vi "LCR_PlotHelper.vi"(5 "Y-Axis":T3, 7 "X-Axis":T3, 9 "Data_IN":T1={"Value"=0.0, "GUI Data Cluster"={"SBR"=0}, "Timing"={"Last Operation"=0.0, "Stop @ T"=FALSE, "Delta T Log"=FALSE, "End T"=0.0, "Delta T"=0.0, "Last Temp"=0.0}, "Measurements"=[], "Hardware"={"VNA TCP Port"=5025, "Global T VAR"="", "Global B VAR"=""}} {"GUI Data Cluster"."SBR" format="%08b"}, 11 "Graph REF":refnum<vi>) -> (0 "Graph Out":cluster{"Variant X":dbl, "Variant Y":dbl}[](array[cluster]), 1 "Data_Out":T1={"Value"=0.0, "GUI Data Cluster"={"SBR"=0}, "Timing"={"Last Operation"=0.0, "Stop @ T"=FALSE, "Delta T Log"=FALSE, "End T"=0.0, "Delta T"=0.0, "Last Temp"=0.0}, "Measurements"=[], "Hardware"={"VNA TCP Port"=5025, "Global T VAR"="", "Global B VAR"=""}} {"GUI Data Cluster"."SBR" format="%08b"})   [LabVIEW 2021]
uses:
  Plotting-Axis.ctl
  Data_Cluster.ctl
  Measurement_Cluster.ctl
  82b2c7e2-1130-4631-9edb-692d0da541f7.vi
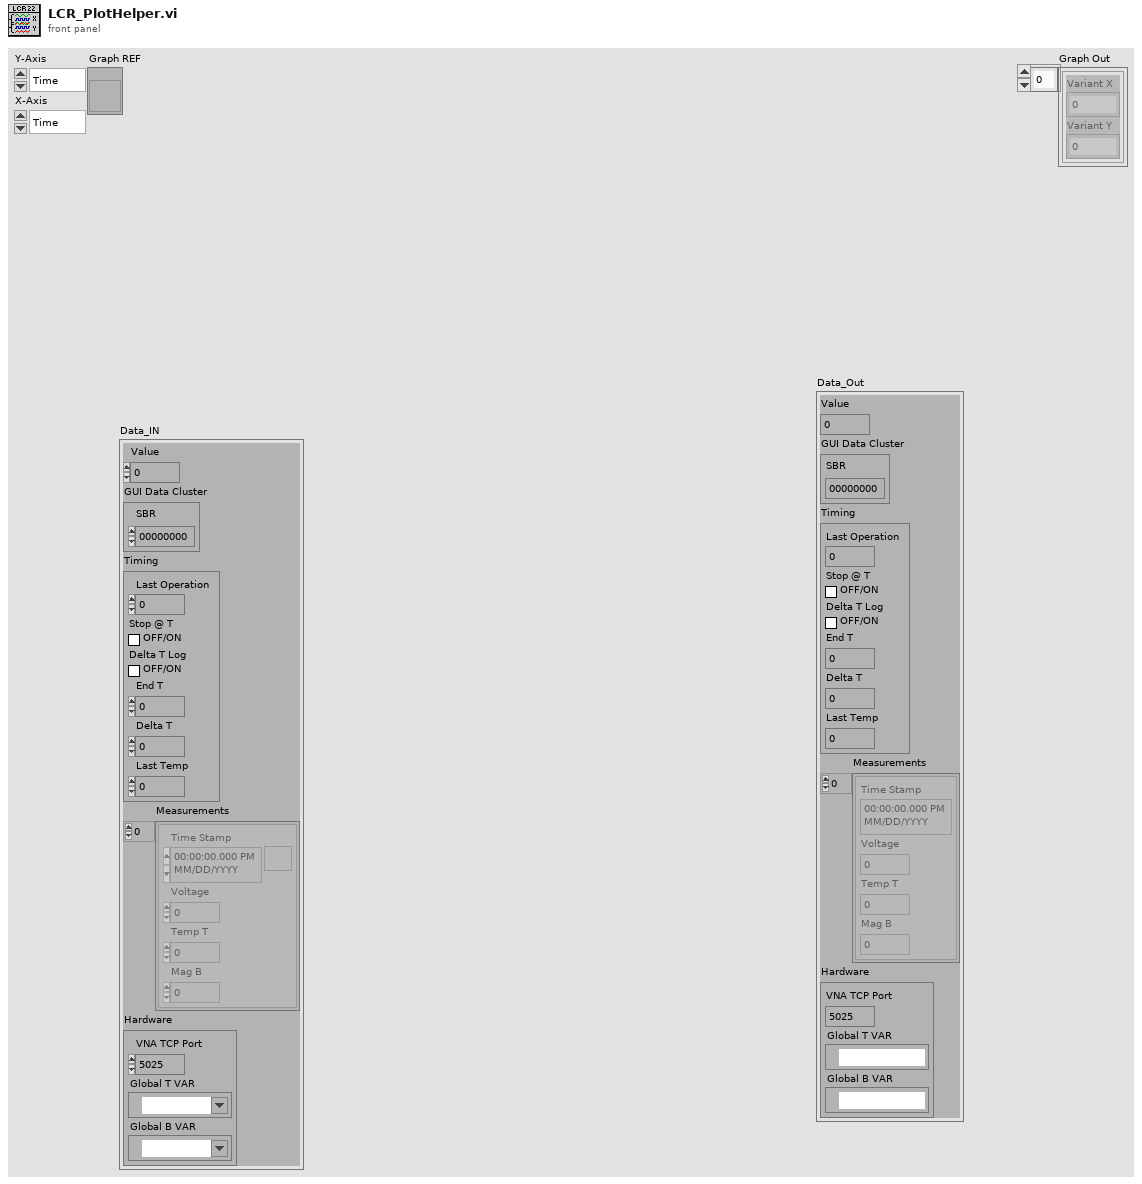
[diagram p1: front panel]
types:
  T1 = typedef "Data_Cluster.ctl" = cluster{"Value":dbl, "GUI Data Cluster":cluster{"SBR":u16}, "Timing":cluster{"Last Operation":dbl, "Stop @ T":bool, "Delta T Log":bool, "End T":dbl, "Delta T":dbl, "Last Temp":dbl}, "Measurements":T2[], "Hardware":cluster{"VNA TCP Port":i32, "Global T VAR":refnum<k21>, "Global B VAR":refnum<k21>}}
  T2 = typedef "Measurement_Cluster.ctl" = cluster{"Time Stamp":timestamp, "Voltage":dbl, "Temp T":dbl, "Mag B":dbl}
  T3 = typedef "Plotting-Axis.ctl" = enum16{"Time", "Temperature A", "Temperature B", "Voltage"}
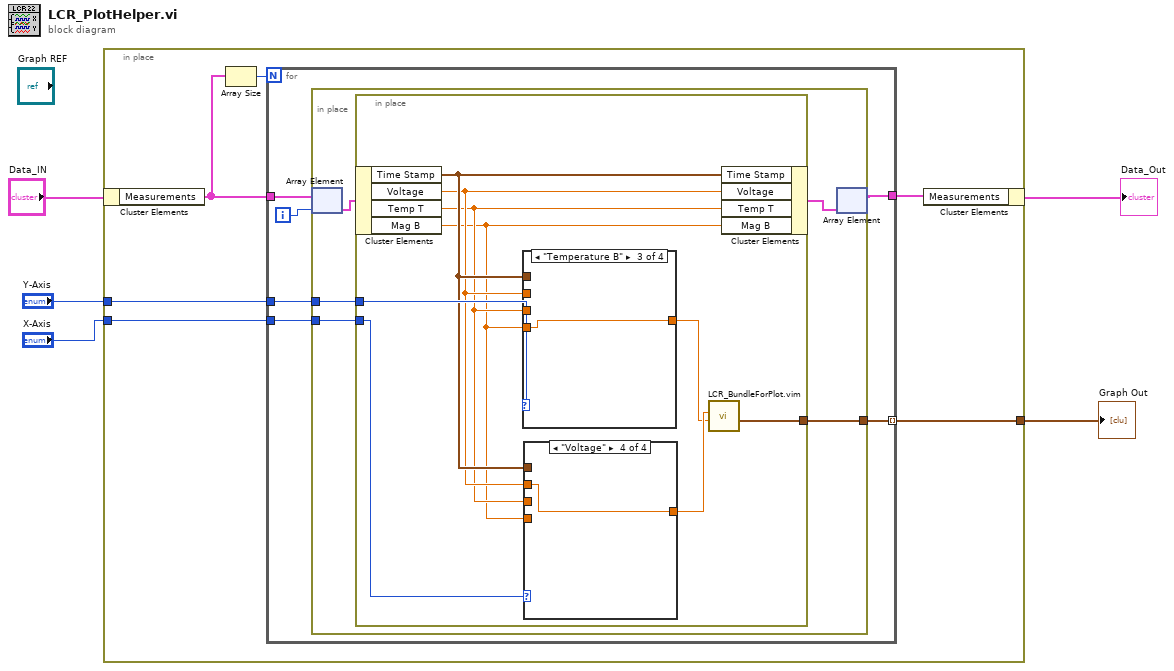
[diagram p0: block diagram]
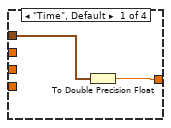
[diagram p2: hidden frame]
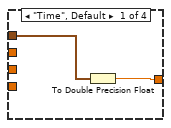
[diagram p5: hidden frame]
diagram:
  n1 = in-place {
    in-place-border: "Y-Axis" -> [w9]
    in-place-border: "X-Axis" -> [w8]
    in-place-border: [w6] -> w1
    n2 = in-place-cluster #1("Data_IN") -> ("Measurements"=w11:T2[])
    n3 = Array Size(array=w11) -> (size(s)=w10:i32)
    n4 = for {
      N: w10 -> [_]
      tunnel: w11 -> [w17]
      tunnel: w9 -> [w15]
      tunnel: w8 -> [w14]
      tunnel: [w13] -> w7
      tunnel: [w12] -> w6 mode=indexing
      i -> [w16]
      n5 = in-place {
        in-place-border: w15 -> [w21]
        in-place-border: w14 -> [w20]
        in-place-border: [w18] -> w12
        n6 = in-place-array #2(w17, w16) -> (w22:T2)
        n7 = in-place {
          in-place-border: w21 -> [w31]
          in-place-border: w20 -> [w30]
          in-place-border: [w23] -> w18
          n8 = in-place-cluster #3(w22) -> ("Time Stamp"=w27:timestamp, "Voltage"=w26:dbl, "Temp T"=w25:dbl, "Mag B"=w24:dbl)
          n9 = case shown="\"Temperature B\"" w31 {
            tunnel: w27 -> [w38 _ _ _]
            tunnel: w26 -> [_ _ _ w41]
            tunnel: w25 -> [_ w39 _ _]
            tunnel: w24 -> [_ _ w40 _]
            tunnel: [w37 w39 w40 w41] -> w28
            frame "Time", Default {
              n10 = To Double Precision Float(number=w38) -> (double precision float=w37:dbl)
            }
            frame "Temperature A" {
            }
            frame "Temperature B" {
            }
            frame "Voltage" {
            }
          }
          n11 = case shown="\"Voltage\"" w30 {
            tunnel: w27 -> [w33 _ _ _]
            tunnel: w26 -> [_ _ _ w36]
            tunnel: w25 -> [_ w34 _ _]
            tunnel: w24 -> [_ _ w35 _]
            tunnel: [w32 w34 w35 w36] -> w29
            frame "Time", Default {
              n12 = To Double Precision Float(number=w33) -> (double precision float=w32:dbl)
            }
            frame "Temperature A" {
            }
            frame "Temperature B" {
            }
            frame "Voltage" {
            }
          }
          n13 = call "LCR_BundleForPlot.vim"("Variant Y"=w28, "Variant X"=w29) -> ("Bundled Variant"=w23:cluster{"Variant X":dbl, "Variant Y":dbl})  [unwired: 9 in]
          n14 = in-place-cluster #3("Time Stamp"=w27, "Voltage"=w26, "Temp T"=w25, "Mag B"=w24) -> (w19:T2)
        }
        n15 = in-place-array #2(w19) -> (w13:T2[])  [unwired: 1 out]
      }
    }
    n16 = in-place-cluster #1("Measurements"=w7) -> (→"Data_Out":T1)
  }
  "Graph Out" <- w1
